vi "Set Filepath.vi"(8 "error in":errorcluster, 10 "Filepath":path, 11 "FileHandler in":refnum<class "NetworkHandler.lvclass">) -> (0 "error out":errorcluster, 3 "FileHandler out":refnum<class "NetworkHandler.lvclass">)   [LabVIEW 2024, in "NetworkHandler.lvclass"]
doc: "____\nHAMPEL SOFTWARE ENGINEERING v2.2.2 (2025-01-16 15:41)"
uses:
  NetworkHandler.lvclass
  NetworkHandler.lvclass/NetworkHandler.ctl
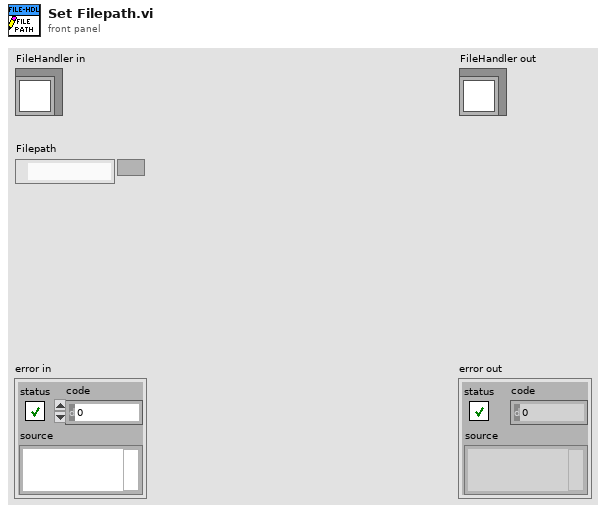
[diagram p1: front panel]
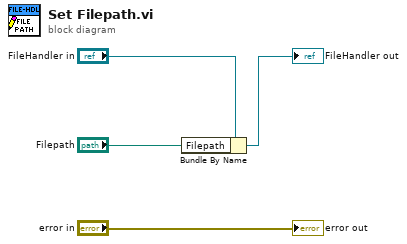
[diagram p0: block diagram]
diagram:
  n1 = Bundle By Name(cluster="FileHandler in", "Filepath"="Filepath") -> (→"FileHandler out":refnum<class "NetworkHandler.lvclass">)
  "error out" <- "error in"
